vi "ViPath.vi"(7 "LabVIEW Web Service Request":refnum<class "Web Request.lvclass">) -> (1 "ApplicationDir":string, 3 "CurrentVIPath":string)   [LabVIEW 2020]
uses:
  <vilib>/wsapi/Web Request.lvclass
panel:
  out "value":string
  # "Use the Web Service Request input terminal to call the VIs on the Web Services palette. Do not remove it from the connector pane unless you don't need access to the palette."
  # "http://127.0.0.1:80/WebService/ViPath"
  # "Each additional control wired to the connector pane will be available as an input in the URL. To include an indicator in terminal-mode output (the default setting), it must also be wired to the connector pane."
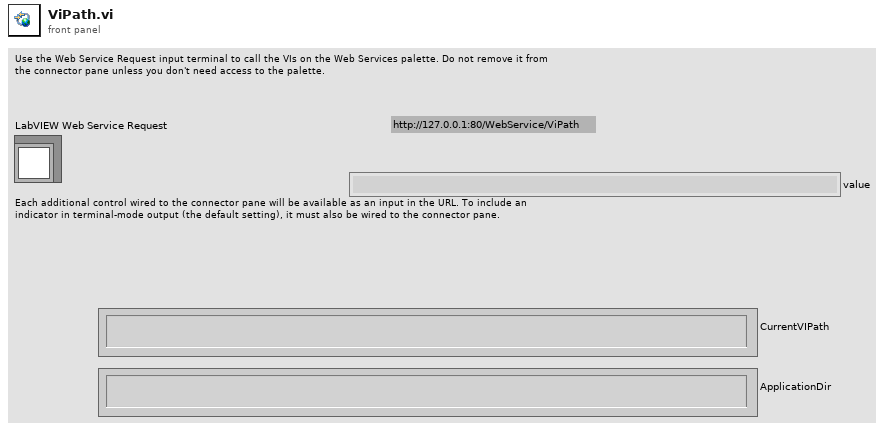
[diagram p1: front panel]
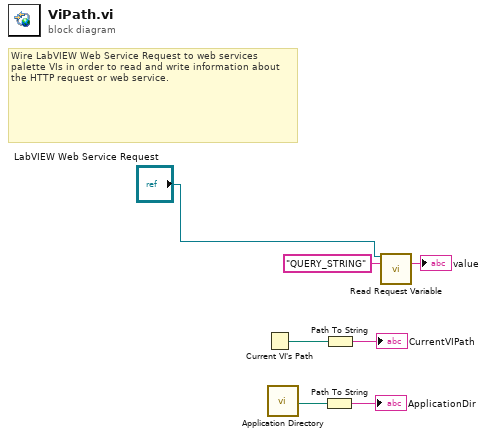
[diagram p0: block diagram]
diagram:
  # "Wire LabVIEW Web Service Request to web services palette VIs in order to read and write information about the HTTP request or web service."
  n1 = Current VI's Path() -> (path=w5:path)
  n2 = call <vilib>:"Application Directory.vi"() -> ("Application Directory"=w2:path)
  n3 = Path To String(path=w2) -> (string=→"ApplicationDir":string)
  n4 = Path To String(path=w5) -> (string=→"CurrentVIPath":string)
  n5 = call <vilib>:"Read Request Variable.vi"("LabVIEW Web Service Request"="LabVIEW Web Service Request", "variable name"="QUERY_STRING") -> ("value"=→"value":string)  [unwired: 11 in, 2 out]
